vi "Display v1.vi"() -> ()   [LabVIEW 2013]
uses:
  Global 1.vi
panel:
  in  "Tab Control":enum32{"Page 1", "Page 2"}(tab)
  out "#1":dbl
  out "#2":dbl
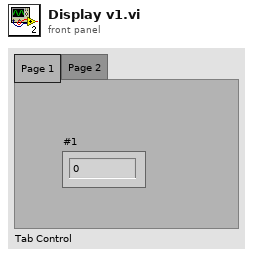
[diagram p1: front panel]
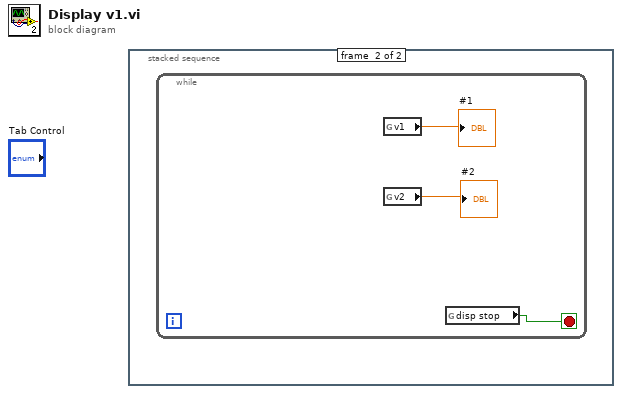
[diagram p0: block diagram]
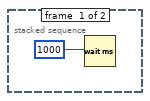
[diagram p2: hidden frame]
diagram:
  n1 = stacked-sequence {
    frame #0 {
      n2 = Wait (ms)(milliseconds to wait=1000) -> ()  [unwired: 1 out]
    }
    frame #1 {
      n3 = while {
        stop <- w2 stop-if-true
        n4 = global read "Global 1.vi" "v1"() -> (→"#1":dbl)
        n5 = global read "Global 1.vi" "v2"() -> (→"#2":dbl)
        n6 = global read "Global 1.vi" "disp stop"() -> (w2:bool)
      }
    }
  }
